vi "Main Search UI.vi"(11 "Startup Notifier":refnum<notifier>) -> ()   [LabVIEW 2016, in "Better Search.lvlib" / "BetterSearch.lvclass"]
uses:
  BetterSearch.lvclass
  Search/Search.lvclass
  Data Types/Search Context.ctl
  Better Search.lvlib
  Data Types/Start Search Type.ctl
  Data Types/Type Reflection Item.ctl
  Data Types/Context Comms.ctl
panel:
  in  "b":bool
  in  "x":bool
  in  "Searches":i32(listbox)
  # "Search History"
  # "To start another search, launch from QuickDrop or a right click search option."
  # "Double-click to discard search"
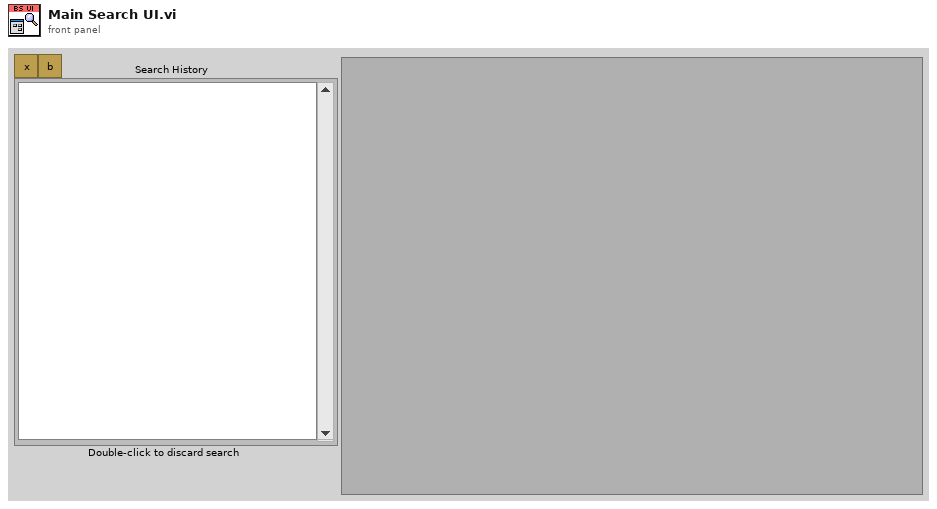
[diagram p1: front panel]
types:
  T1 = typedef "Better Search.lvlib/BetterSearch.lvclass/Main Events.ctl" = cluster{"Context":refnum<user-event>, "Start Search":refnum<user-event>, "New Result":refnum<user-event>, "Dim UI":refnum<user-event>, "Close":refnum<user-event>, "Progress WD":refnum<user-event>}
  T2 = typedef "Better Search.lvlib/Search Context.ctl" = cluster{"Type ID":string, "VI Refnum":refnum<vi>, "Starting Text":string, "Shift?":bool, "App Ref":refnum<vi>, "Start Search Type":T3, "Item Graph":T4[], "Variant":variant}
  T3 = typedef "Better Search.lvlib/Start Search Type.ctl" = enum16{"Auto", "Text", "Data Type", "Bundle"}
  T4 = typedef "Better Search.lvlib/Type Reflection Item.ctl" = cluster{"Parent":i32, "Depth":i32, "Children":i32[], "Skip":bool, "Name":string, "Type":variant, "TypeID":string}
  T5 = enum32{"Invalid", "Standard", "Closed", "Hidden", "Minimized", "Maximized"}
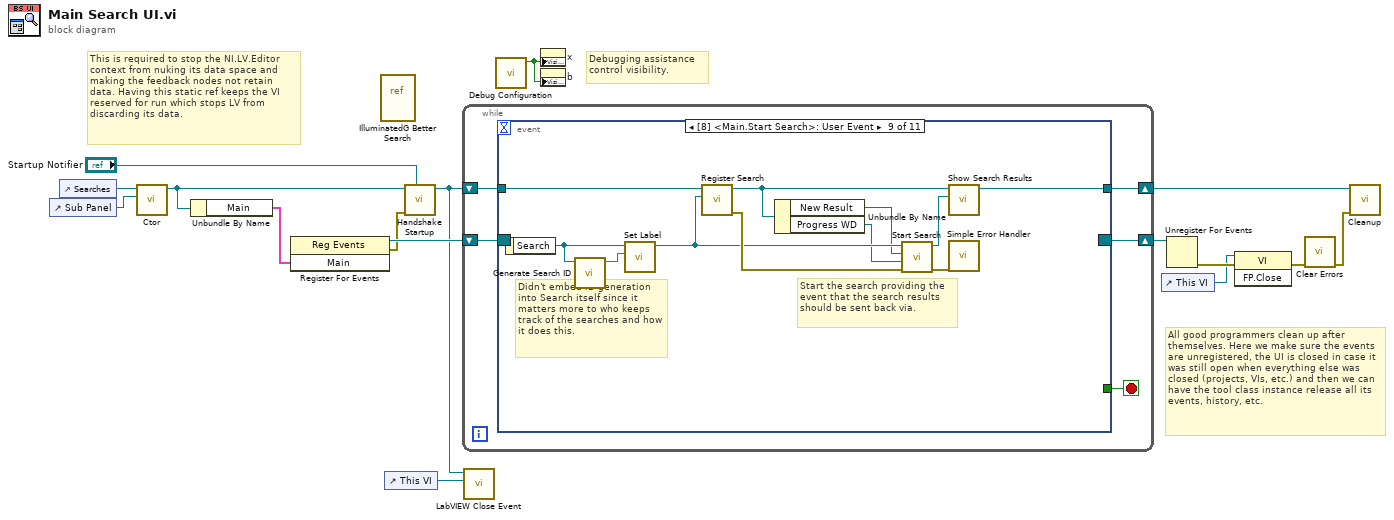
[diagram p0: block diagram]
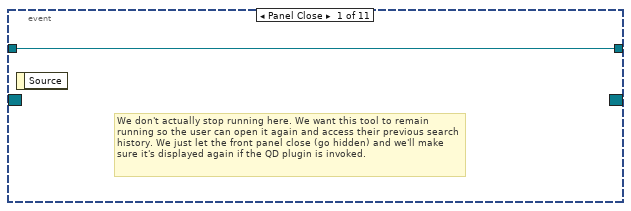
[diagram p2: hidden frame]
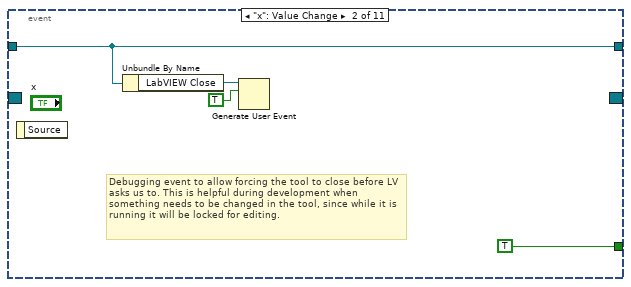
[diagram p3: hidden frame]
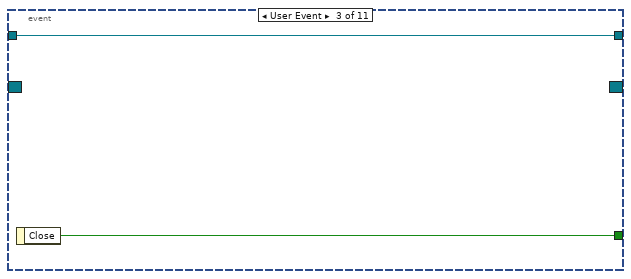
[diagram p4: hidden frame]
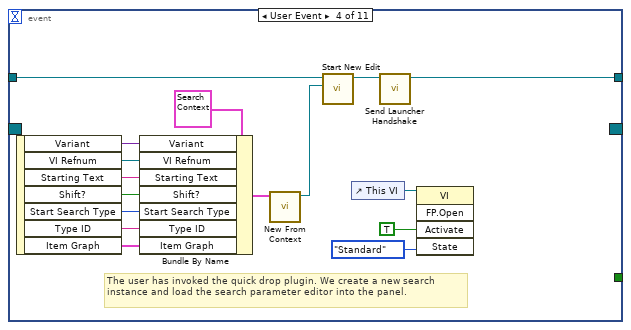
[diagram p5: hidden frame]
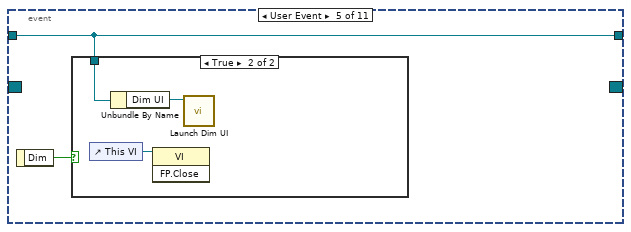
[diagram p6: hidden frame]
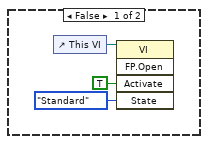
[diagram p7: hidden frame]
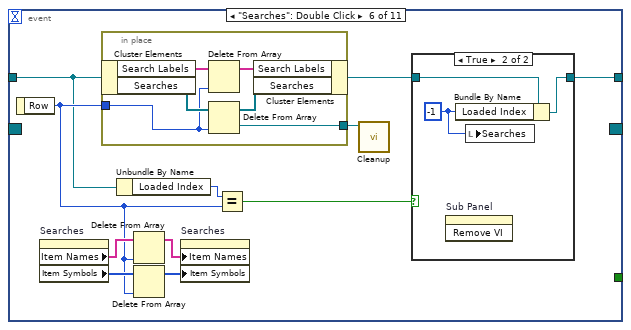
[diagram p8: hidden frame]
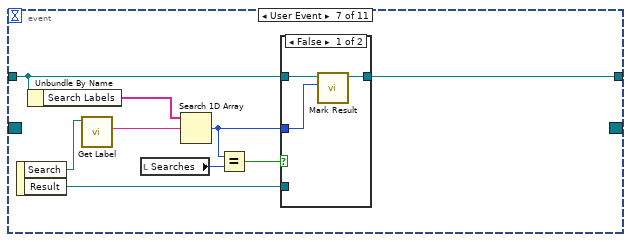
[diagram p10: hidden frame]
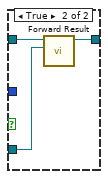
[diagram p11: hidden frame]
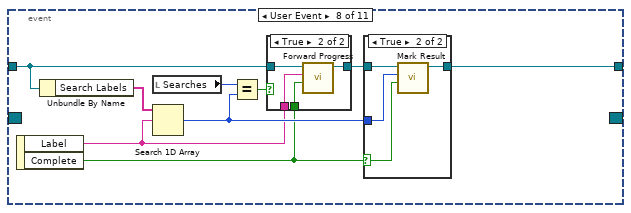
[diagram p12: hidden frame]
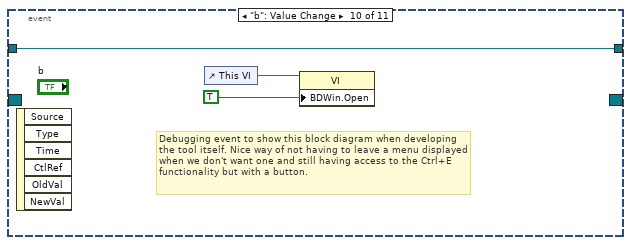
[diagram p15: hidden frame]
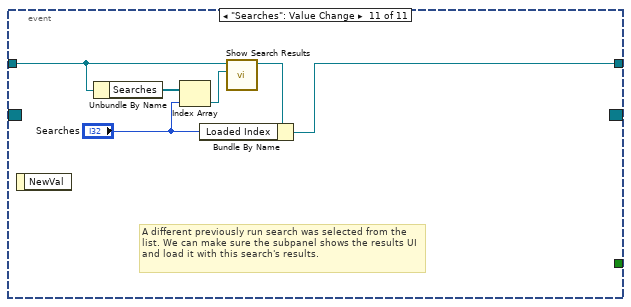
[diagram p16: hidden frame]
diagram:
  # "Debugging assistance control visibility."
  # "All good programmers clean up after themselves. Here we make sure the events are unregistered, the UI is closed in case it was still open when everything else was closed (projects, VIs, etc.) and then we can have the tool class instance release all its events, history, etc."
  # "This is required to stop the NI.LV.Editor context from nuking its data space and making the feedback nodes not retain data. Having this static ref keeps the VI reserved for run which stops LV from discarding its data."
  n1 = control-ref of="Sub Panel"() -> (w14:refnum<vi>)
  n2 = control-ref of="Searches"() -> (w15:refnum<vi>)
  n3 = call "Ctor.vi"("Panel Ref"=w14, "List Ref"=w15) -> ("BetterSearch out"=w3:refnum<class "BetterSearch.lvclass">)  [unwired: 8 in, 1 out]
  n4 = Unbundle By Name(w3) -> ("Main"=w2:T1)
  n5 = register-events(w2) -> (reference out=w11:refnum<event-registration>, error out=w7:errorcluster)  [unwired: 2 in]
  n6 = vi-ref "IlluminatedG Better Search.vi"() -> ()  [unwired: 1 out]
  n7 = control-ref of="This VI"() -> (w1:refnum<vi>)
  n8 = call "Handshake Startup.vi"("Startup Notifier"="Startup Notifier", "error in (no error)"=w7, "BetterSearch in"=w3) -> ("BetterSearch out"=w4:refnum<class "BetterSearch.lvclass">)  [unwired: 7 in, 1 out]
  n9 = while {
    shift-right: [w20] -> w16
    shift-left: w11 -> [w21]
    shift-right: [w17] -> w10
    shift-left: w4 -> [w18]
    stop <- w19 stop-if-true
    n10 = event shown="[8] <Main.Start Search>: User Event" {
      selector: w21 -> [_ _ _ _ _ _ _ _ _ _ _]
      dyn-events: [_ _ _ _ _ _ _ _ _ _ _] -> w20
      timeout: _ -> [_ _ _ _ _ _ _ _ _ _ _]
      tunnel: [_ TRUE ("Close") w27 _ _ _ _ _ _ _ _] -> w19
      tunnel: w18 -> [w22 w26 w28 w32 w45 w53 w77 w92 w115 w121 w126]
      tunnel: [w22 w26 w28 w33 w45 w55 w75 w96 w111 w121 w123] -> w17
      event Panel Close {
        # "We don't actually stop running here. We want this tool to remain running so the user can open it again and access their previous search history. We just let the front panel close (go hidden) and we'll make sure it's displayed again if the QD plugin is invoked."
        n11 = event-data() -> ()  [unwired: 1 in, 1 out]
      }
      event "x": Value Change {
        # "Debugging event to allow forcing the tool to close before LV asks us to. This is helpful during development when something needs to be changed in the tool, since while it is running it will be locked for editing."
        n12 = event-data() -> ()  [unwired: 1 in, 1 out]
        n13 = Unbundle By Name(w26) -> ("LabVIEW Close"=w25:refnum<user-event>)
        n14 = Generate User Event(user event=w25, event data cluster=TRUE ("event data")) -> ()  [unwired: 2 in, 2 out]
      }
      event User Event {
        n15 = event-data() -> ("Close"=w27:bool)  [unwired: 1 in]
      }
      event User Event {
        # "The user has invoked the quick drop plugin. We create a new search instance and load the search parameter editor into the panel."
        n16 = event-data() -> ("Variant"=w40:variant, "VI Refnum"=w39:refnum<vi>, "Starting Text"=w38:string, "Shift?"=w37:bool, "Start Search Type"=w31:T3, "Type ID"=w30:string, "Item Graph"=w29:T4[])  [unwired: 1 in]
        n17 = Bundle By Name(cluster=T2 {"Type ID"="", "VI Refnum"=refnum, "Starting Text"="", "Shift?"=FALSE, "App Ref"=refnum, "Start Search Type"=enum."Auto", "Item Graph"=[], "Variant"=variant} ("Search Context"), "Variant"=w40, "VI Refnum"=w39, "Starting Text"=w38, "Shift?"=w37, "Start Search Type"=w31, "Type ID"=w30, "Item Graph"=w29) -> (w36:T2)
        n18 = call "New From Context.vi"("Search Context"=w36) -> ("Search out"=w35:refnum<class "Search.lvclass">)  [unwired: 9 in, 1 out]
        n19 = call "Start New Edit.vi"("New Search"=w35, "BetterSearch in"=w32) -> ("BetterSearch out"=w34:refnum<class "BetterSearch.lvclass">)  [unwired: 8 in, 1 out]
        n20 = control-ref of="This VI"() -> (w44:refnum<vi>)
        n21 = call "Send Launcher Handshake.vi"("BetterSearch in"=w34) -> ("BetterSearch out"=w33:refnum<class "BetterSearch.lvclass">)  [unwired: 9 in, 1 out]
        n22 = invoke class="VI" method="FP.Open"(reference=w44, "Activate"=TRUE ("Activate?"), "State"=T5."Standard") -> ()  [unwired: 2 in, 5 out]
      }
      event User Event {
        n23 = event-data() -> ("Dim"=w46:bool)  [unwired: 1 in]
        n24 = case shown="True" w46 {
          tunnel: w45 -> [_ w51]
          frame False {
            n25 = control-ref of="This VI"() -> (w49:refnum<vi>)
            n26 = invoke class="VI" method="FP.Open"(reference=w49, "Activate"=TRUE ("Activate?"), "State"=T5."Standard") -> ()  [unwired: 2 in, 5 out]
          }
          frame True {
            n27 = control-ref of="This VI"() -> (w52:refnum<vi>)
            n28 = Unbundle By Name(w51) -> ("Dim UI"=w50:refnum<user-event>)
            n29 = invoke class="VI" method="FP.Close"(reference=w52) -> ()  [unwired: 2 in, 3 out]
            n30 = call "Launch Dim UI.vi"("Dim UI"=w50) -> ()  [unwired: 11 in]
          }
        }
      }
      event "Searches": Double Click {
        n31 = event-data() -> ("Row"=w54:i32)  [unwired: 1 in]
        n32 = property on="Searches" class="LstBox (strict)"() -> ("Item Names"=w61:string[], "Item Symbols"=w62:i32[])  [unwired: 2 in, 2 out]
        n33 = in-place {
          in-place-border: w54 -> [w68]
          in-place-border: [w71] -> w63
          n34 = in-place-cluster #1(w53) -> ("Search Labels"=w70:string[], "Searches"=w73:refnum<class "Search.lvclass">[])
          n35 = Delete From Array(array=w70, index=w68) -> (array with subset deleted=w69:string[])  [unwired: 1 in, 1 out]
          n36 = Delete From Array(array=w73, index=w68) -> (deleted portion=w71:refnum<class "Search.lvclass">, array with subset deleted=w72:refnum<class "Search.lvclass">[])  [unwired: 1 in]
          n37 = in-place-cluster #1("Search Labels"=w69, "Searches"=w72) -> (w56:refnum<class "BetterSearch.lvclass">)
        }
        n38 = Unbundle By Name(w53) -> ("Loaded Index"=w58:i32)
        n39 = Delete From Array(array=w61, index=w54) -> (array with subset deleted=w59:string[])  [unwired: 1 in, 1 out]
        n40 = Delete From Array(array=w62, index=w54) -> (array with subset deleted=w60:i32[])  [unwired: 1 in, 1 out]
        n41 = property on="Searches" class="LstBox (strict)"("Item Names"=w59, "Item Symbols"=w60) -> ()  [unwired: 2 in, 2 out]
        n42 = Equal?(x=w58, y=w54) -> (x = y?=w57:bool)
        n43 = call "Cleanup.vi"("Search in"=w63) -> ()  [unwired: 10 in, 1 out]
        n44 = case shown="True" w57 {
          tunnel: w56 -> [w64 w67]
          tunnel: [w64 w66] -> w55
          frame False {
          }
          frame True {
            w65 = -1 ("Loaded Index")
            n45 = invoke on="Sub Panel" class="SubPnl" method="Remove VI"() -> ()  [unwired: 3 in, 3 out]
            n46 = Bundle By Name(cluster=w67, "Loaded Index"=w65) -> (w66:refnum<class "BetterSearch.lvclass">)
            n47 = local write "Searches"(w65) -> ()
          }
        }
      }
      event User Event {
        n48 = event-data() -> ("Search"=w82:refnum<class "Search.lvclass">, "Result"=w76:refnum<class "Search Result.lvclass">)  [unwired: 1 in]
        n49 = Unbundle By Name(w77) -> ("Search Labels"=w81:string[])
        n50 = call "Get Label.vi"("Search in"=w82) -> ("Label"=w80:string)  [unwired: 8 in, 2 out]
        n51 = local read "Searches"() -> (w79:i32)
        n52 = Search 1D Array(1D array=w81, element=w80) -> (index of element=w74:i32)  [unwired: 1 in]
        n53 = Equal?(x=w74, y=w79) -> (x = y?=w78:bool)
        n54 = case shown="False" w78 {
          tunnel: w77 -> [w85 w88]
          tunnel: w76 -> [_ w87]
          tunnel: [w84 w86] -> w75
          tunnel: w74 -> [w83 _]
          frame False {
            n55 = call "Mark Result.vi"("Search Index"=w83, "BetterSearch in"=w85) -> ("BetterSearch out"=w84:refnum<class "BetterSearch.lvclass">)  [unwired: 8 in, 1 out]
          }
          frame True {
            n56 = call "Forward Result.vi"("Result"=w87, "BetterSearch in"=w88) -> ("BetterSearch out"=w86:refnum<class "BetterSearch.lvclass">)  [unwired: 8 in, 1 out]
          }
        }
      }
      event User Event {
        n57 = event-data() -> ("Label"=w90:string, "Complete"=w89:bool)  [unwired: 1 in]
        n58 = Unbundle By Name(w92) -> ("Search Labels"=w97:string[])
        n59 = local read "Searches"() -> (w95:i32)
        n60 = Search 1D Array(1D array=w97, element=w90) -> (index of element=w94:i32)  [unwired: 1 in]
        n61 = Equal?(x=w95, y=w94) -> (x = y?=w93:bool)
        n62 = case shown="True" w93 {
          tunnel: w92 -> [w98 w102]
          tunnel: [w98 w101] -> w91
          tunnel: w90 -> [_ w100]
          tunnel: w89 -> [_ w99]
          frame False {
          }
          frame True {
            n63 = call "Forward Progress.vi"("Complete"=w99, "Search Label"=w100, "BetterSearch in"=w102) -> ("BetterSearch out"=w101:refnum<class "BetterSearch.lvclass">)  [unwired: 7 in, 1 out]
          }
        }
        n64 = case shown="True" w89 {
          selector: w89 -> [_ w104]
          tunnel: w91 -> [w103 w107]
          tunnel: [w103 w106] -> w96
          tunnel: w94 -> [_ w105]
          frame False {
          }
          frame True {
            n65 = call "Mark Result.vi"("Complete (F)"=w104, "Search Index"=w105, "BetterSearch in"=w107) -> ("BetterSearch out"=w106:refnum<class "BetterSearch.lvclass">)  [unwired: 7 in, 1 out]
          }
        }
      }
      event User Event {
        # "Start the search providing the event that the search results should be sent back via."
        # "Didn't embed ID generation into Search itself since it matters more to who keeps track of the searches and how it does this."
        n66 = event-data() -> ("Search"=w117:refnum<class "Search.lvclass">)  [unwired: 1 in]
        n67 = call "Generate Search ID.vi"("Search"=w117) -> ("Search ID"=w116:string)  [unwired: 10 in]
        n68 = call "Set Label.vi"("Label"=w116, "Search in"=w117) -> ("Search out"=w114:refnum<class "Search.lvclass">)  [unwired: 8 in, 1 out]
        n69 = call "Register Search.vi"("Search"=w114, "BetterSearch in"=w115) -> ("error out"=w118:errorcluster, "BetterSearch out"=w112:refnum<class "BetterSearch.lvclass">)  [unwired: 8 in]
        n70 = Unbundle By Name(w112) -> ("New Result"=w113:refnum<user-event>, "Progress WD"=w108:refnum<user-event>)
        n71 = call "Start Search.vi"("error in (no error)"=w118, "Progress WD"=w108, "New Result Event"=w113, "Search in"=w114) -> ("error out"=w109:errorcluster, "Search out"=w110:refnum<class "Search.lvclass">)  [unwired: 6 in]
        n72 = call "Show Search Results.vi"("Search"=w110, "BetterSearch in"=w112) -> ("BetterSearch out"=w111:refnum<class "BetterSearch.lvclass">)  [unwired: 8 in, 1 out]
        n73 = call <vilib>:"Simple Error Handler.vi"("error in (no error)"=w109) -> ()  [unwired: 4 in, 5 out]
      }
      event "b": Value Change {
        # "Debugging event to show this block diagram when developing the tool itself. Nice way of not having to leave a menu displayed when we don't want one and still having access to the Ctrl+E functionality but with a button."
        n74 = event-data() -> ()  [unwired: 1 in, 6 out]
        n75 = control-ref of="This VI"() -> (w120:refnum<vi>)
        n76 = property class="VI"(reference=w120, "BDWin.Open"=TRUE ("Block Diagram Window:Open")) -> ()  [unwired: 1 in, 2 out]
      }
      event "Searches": Value Change {
        # "A different previously run search was selected from the list. We can make sure the subpanel shows the results UI and load it with this search's results."
        n77 = event-data() -> ()  [unwired: 1 in, 1 out]
        n78 = Unbundle By Name(w126) -> ("Searches"=w127:refnum<class "Search.lvclass">[])
        n79 = Index Array(array=w127, index="Searches") -> (element=w125:refnum<class "Search.lvclass">)
        n80 = call "Show Search Results.vi"("Search"=w125, "BetterSearch in"=w126) -> ("BetterSearch out"=w124:refnum<class "BetterSearch.lvclass">)  [unwired: 8 in, 1 out]
        n81 = Bundle By Name(cluster=w124, "Loaded Index"="Searches") -> (w123:refnum<class "BetterSearch.lvclass">)
      }
    }
  }
  n82 = call "LabVIEW Close Event.vi"("VI Refnum"=w1, "BetterSearch"=w4) -> ()  [unwired: 10 in]
  n83 = call "Debug Configuration.vi"() -> ("Flag?"=w5:bool)  [unwired: 11 in]
  n84 = property on="x" class="Bool"("Visible"=w5) -> ()  [unwired: 2 in, 2 out]
  n85 = property on="b" class="Bool"("Visible"=w5) -> ()  [unwired: 2 in, 2 out]
  n86 = control-ref of="This VI"() -> (w12:refnum<vi>)
  n87 = Unregister For Events(event registration refnum=w16) -> (error out=w13:errorcluster)  [unwired: 1 in]
  n88 = invoke class="VI" method="FP.Close"(reference=w12, error in=w13) -> (error out=w9:errorcluster)  [unwired: 1 in, 2 out]
  n89 = call <vilib>:"Clear Errors.vi"("error in (no error)"=w9) -> ("error out"=w8:errorcluster)  [unwired: 5 in, 1 out]
  n90 = call "Cleanup.vi"("error in (no error)"=w8, "BetterSearch in"=w10) -> ()  [unwired: 9 in, 1 out]
